vi "myXi_GetDataFrameStats.vi"(8 "error in (no error)":errorcluster, 11 "xiCam IN":refnum<k24>) -> (0 "error out":errorcluster, 2 "skipped frame":T1, 3 "xiCam Out":refnum<k24>)   [LabVIEW 2018]
uses:
  C:/XIMEA/API/x64/xiApi.NETX64.dll
  VisionLibrariesXimea/xiLib/xiLIB_64bit/xiLIB/xiCamLib/xiCam/PRM/PRM/PRM_v2.ctl
  VisionLibrariesXimea/xiLib/xiLIB_64bit/xiLIB/xiCamLib/xiCam/PRM/COUNTER_SELECTOR/COUNTER_SELECTOR.ctl
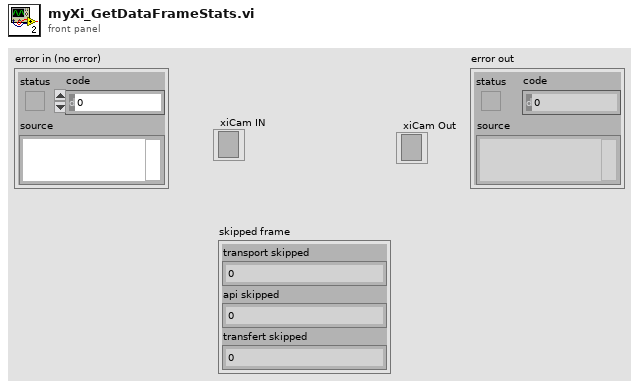
[diagram p1: front panel]
types:
  T1 = cluster{"transport skipped":i32, "api skipped":i32, "transfert skipped":i32}
  T2 = typedef "COUNTER_SELECTOR.ctl" = enum16{"CNT_SEL_TRANSPORT_SKIPPED_FRAMES", "CNT_SEL_API_SKIPPED_FRAMES", "CNT_SEL_TRANSPORT_TRANSFERRED_FRAMES"}
  T3 = typedef "PRM_v2.ctl" = enum16{"ACQ_BUFFER_SIZE", "ACQ_FRAME_BURST_COUNT", "ACQ_TIMING_MODE", "ACQ_TRANSPORT_BUFFER_SIZE", "AE_MAX_LIMIT", "AEAG", "AEAG_LEVEL", "API_VERSION", "AG_MAX_LIMIT", "APPLY_CMS", "AUTO_BANDWIDTH_CALCULATION", "AUTO_WB", "AVAILABLE_BANDWIDTH", "AVAILABLE_BANDWIDTH_MAX", "AVAILABLE_BANDWIDTH_MIN", "BPC", "BUFFER_POLICY", "BUFFERS_QUEUE_SIZE", "CC_MATRIX_00", "CC_MATRIX_01", "CC_MATRIX_02", "CC_MATRIX_03", "CC_MATRIX_10", "CC_MATRIX_11", "CC_MATRIX_12", "CC_MATRIX_13", "CC_MATRIX_20", "CC_MATRIX_21", "CC_MATRIX_22", "CC_MATRIX_23", "CC_MATRIX_30", "CC_MATRIX_31", "CC_MATRIX_32", "CC_MATRIX_33", "CHIP_TEMP", "CMS", "COLOR_FILTER_ARRAY", "COOLING", "DEBOUNCE_EN", "DEBOUNCE_POL", "DEBOUNCE_T0", "DEBOUNCE_T1", "DEBUG_LEVEL", "DEFAULT_CC_MATRIX", "DEVICE_INSTANCE_PATH", "DEVICE_MODEL_ID", "DEVICE_NAME", "DEVICE_SN", "DEVICE_TYPE", "DEVICE_USER_ID", "DOWNSAMPLING", "DOWNSAMPLING_MAX", "DOWNSAMPLING_MIN", "DOWNSAMPLING_TYPE", "DRV_VERSION", "EXP_PRIORITY", "EXPOSURE", "EXPOSURE_DIRECT_UPDATE", "EXPOSURE_MAX", "EXPOSURE_MIN", "FFS_FILE_NAME", "FPGA1_VERSION", "FRAMERATE", "FRAMERATE_MAX", "FRAMERATE_MIN", "FREE_FFS_SIZE", "GAIN", "GAIN_DIRECT_UPDATE", "GAIN_MAX", "GAIN_MIN", "GAMMAC", "GAMMAY", "GPI_LEVEL", "GPI_MODE", "GPI_SELECTOR", "GPI_SELECTOR_MAX", "GPI_SELECTOR_MIN", "GPO_MODE", "GPO_SELECTOR", "GPO_SELECTOR_MAX", "GPO_SELECTOR_MIN", "HDR", "HDR_T1", "HDR_T2", "HEIGHT", "HEIGHT_MAX", "HEIGHT_MIN", "HOUSE_TEMP", "IMAGE_DATA_FORMAT", "IMAGE_IS_COLOR", "INPUT_CMS_PROFILE", "IS_COOLED", "IS_DEVICE_EXIST", "KNEEPOINT1", "KNEEPOINT2", "LED_MODE", "LED_SELECTOR", "LED_SELECTOR_MAX", "LED_SELECTOR_MIN", "LIMIT_BANDWIDTH", "LIMIT_BANDWIDTH_MAX", "LIMIT_BANDWIDTH_MIN", "LUT_EN", "LUT_INDEX", "LUT_INDEX_MAX", "LUT_INDEX_MIN", "LUT_VALUE", "LUT_VALUE_MAX", "LUT_VALUE_MIN", "MANUAL_WB", "MCU1_VERSION", "MCU2_VERSION", "OFFSET_X", "OFFSET_X_MAX", "OFFSET_X_MIN", "OFFSET_Y", "OFFSET_Y_MAX", "OFFSET_Y_MIN", "OUTPUT_CMS_PROFILE", "OUTPUT_DATA_BIT_DEPTH", "OUTPUT_DATA_PACKING", "READ_FILE_FFS", "RECENT_FRAME", "SENSOR_DATA_BIT_DEPTH", "SENSOR_MODE", "SENSOR_TAPS", "SHARPNESS", "SHUTTER_TYPE", "TARGET_TEMP", "TRG_DELAY", "TRG_SELECTOR", "TRG_SOFTWARE", "TRG_SOURCE", "USED_FFS_SIZE", "WB_KB", "WB_KG", "WB_KR", "WIDTH", "WIDTH_MAX", "WIDTH_MIN", "WRITE_FILE_FFS", "ACQ_BUFFER_SIZE_UNIT", "ACQ_TRANSPORT_BUFFER_COMMIT", "AEAG_ROI_HEIGHT", "AEAG_ROI_OFFSET_X", "AEAG_ROU_OFFSET_Y", "AEAG_ROI_WIDTH", "API_CONTEXT_LIST", "BINNING_HORIZONTAL", "BINNING_SELECTOR", "BINNING_VERTICAL", "COLUMN_FPN_CORRECTION", "COUNTER_SELECTOR", "COUNTER_VALUE", "DECIMATION_HORIZONTAL", "DECIMATION_SELECTOR", "DECIMATION_VERTICAL", "DEVICE_ID", "DEVICE_LOCATION_PATH", "DEVICE_MANIFEST", "DEVICE_RESET", "DEVICE_SENS_SN", "EXPOSURE_BURST_COUNT", "FFS_ACCESS_KEY", "GAIN_SELECTOR", "HW_REVISION", "IMAGE_BLACK_LEVEL", "IMAGE_DATA_BIT_DEPTH", "IMAGE_DATA_FORMAT_RGB32_ALPHA", "IMAGE_PAYLOAD_SIZE", "LENS_APERTURE_VALUE", "LENS_FEATURE", "LENS_FEATURE_SELECTOR", "LENS_FOCAL_LENGTH", "LENS_FOCUS_DISTANCE", "LENS_FOCUS_MOVE", "LENS_FOCUS_MOVEMENT_VALUE", "LENS_MODE", "OUTPUT_DATA_PACKING_TYPE", "SENSOR_CLOCK_FREQ_HZ", "SENSOR_CLOCK_FREQ_INDEX", "SENSOR_FEATURE_SELECTOR", "SENSOR_FEATURE_VALUE", "SENSOR_OUTPUT_CHANNEL_COUNT", "TRANSPORT_PIXEL_FORMAT", "TS_RST_MODE", "TS_RST_SOURCE"}
  T4 = cluster{"Int32_Value":i32, "Int32_Value":i32, "Int32_Value":i32}
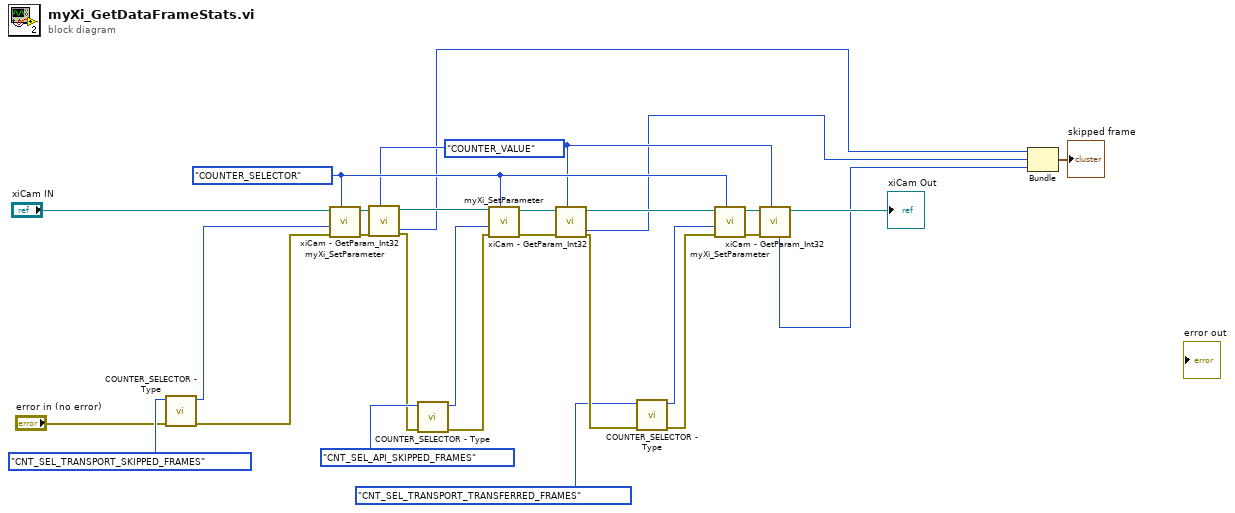
[diagram p0: block diagram]
diagram:
  w7 = PRM_v2."COUNTER_VALUE" ("PRM")
  w8 = PRM_v2."COUNTER_SELECTOR" ("input PRM")
  n1 = call "COUNTER_SELECTOR - Type.vi"("error in (no error)"="error in (no error)", "COUNTER_SELECTOR"=COUNTER_SELECTOR."CNT_SEL_TRANSPORT_SKIPPED_FRAMES") -> ("error out"=w23:errorcluster, "COUNTER_SELECTOR_VALUE"=w1:i32)  [unwired: 8 in]
  n2 = call "myXi_SetParameter.vi"("input PRM"=w8, "error in"=w23, "input value I32"=w1, "xiCam IN"="xiCam IN") -> ("error out"=w27:errorcluster, "xiCam Out"=w25:refnum<k24>)  [unwired: 6 in]
  n3 = call "xiCam - GetParam_Int32.vi"("PRM"=w7, "error in (no error)"=w27, "xiCam In"=w25) -> ("error out"=w20:errorcluster, "xiCam Out"=w21:refnum<k24>, "Int32_Value"=w5:i32)  [unwired: 6 in]
  n4 = call "COUNTER_SELECTOR - Type.vi"("error in (no error)"=w20, "COUNTER_SELECTOR"=COUNTER_SELECTOR."CNT_SEL_API_SKIPPED_FRAMES") -> ("error out"=w19:errorcluster, "COUNTER_SELECTOR_VALUE"=w18:i32)  [unwired: 8 in]
  n5 = call "myXi_SetParameter.vi"("input PRM"=w8, "error in"=w19, "input value I32"=w18, "xiCam IN"=w21) -> ("error out"=w17:errorcluster, "xiCam Out"=w16:refnum<k24>)  [unwired: 6 in]
  n6 = call "xiCam - GetParam_Int32.vi"("PRM"=w7, "error in (no error)"=w17, "xiCam In"=w16) -> ("error out"=w15:errorcluster, "xiCam Out"=w12:refnum<k24>, "Int32_Value"=w4:i32)  [unwired: 6 in]
  n7 = call "COUNTER_SELECTOR - Type.vi"("error in (no error)"=w15, "COUNTER_SELECTOR"=COUNTER_SELECTOR."CNT_SEL_TRANSPORT_TRANSFERRED_FRAMES") -> ("error out"=w10:errorcluster, "COUNTER_SELECTOR_VALUE"=w9:i32)  [unwired: 8 in]
  n8 = call "myXi_SetParameter.vi"("input PRM"=w8, "error in"=w10, "input value I32"=w9, "xiCam IN"=w12) -> ("error out"=w14:errorcluster, "xiCam Out"=w13:refnum<k24>)  [unwired: 6 in]
  n9 = call "xiCam - GetParam_Int32.vi"("PRM"=w7, "error in (no error)"=w14, "xiCam In"=w13) -> ("xiCam Out"=→"xiCam Out":refnum<k24>, "Int32_Value"=w3:i32)  [unwired: 6 in, 1 out]
  n10 = Bundle("Int32_Value"=w5, "Int32_Value"=w4, "Int32_Value"=w3) -> (→"skipped frame":T4)  [unwired: 1 in]
